vi "Unreserve.vi"(0 "SLSC Remote in":refnum<class "SLSC Remote.lvclass">, 5 "devices":refnum<k21>="$DefaultDevices", 11 "error in (no error)":errorcluster) -> (4 "SLSC Remote out":refnum<class "SLSC Remote.lvclass">, 15 "error out":errorcluster)   [LabVIEW 2016, in "SLSC Interfaces.lvlib" / "SLSC Remote.lvclass"]
uses:
  SLSC Remote.lvclass
  C:/Users/tblair/Documents/Git Projects/SLSC-Interface/Source/SLSC Interface Class/SLSC Interface.lvclass
  <vilib>/NI/JSON Support for LabVIEW/JSON Data Classes/JSON Object/JSON Object.lvclass
  C:/Program Files (x86)/National Instruments/LabVIEW 2016/vi.lib/NI/JSON Support for LabVIEW/JSON Data Classes/JSON Datatype/JSON Null.lvclass
  <vilib>/NI/JSON Support for LabVIEW/JSON Data Classes/JSON Object/New JSON Object (Empty).vi
  <vilib>/NI/JSON Support for LabVIEW/JSON Data Classes/JSON Object/Insert Key Value Pair (Single String).vi
  <vilib>/NI/NI JSONRPC Server Framework/Classes/Server/Format Client Request (Auto-Increment).vi
  <vilib>/httpClient/POSTBuffer.vi
  <vilib>/NI/NI JSONRPC Server Framework/Classes/Server/Parse Response (Object).vi
  <vilib>/NI/NI JSONRPC Server Framework/Classes/Server/JSONRPC Server.lvclass
  <vilib>/httpClient/LabVIEWHTTPClient.lvlib
  <vilib>/NI/JSON Support for LabVIEW/JSON Data Classes/JSON Helper/JSON Helper.lvclass
  C:/Program Files (x86)/National Instruments/LabVIEW 2016/vi.lib/NI/JSON Support for LabVIEW/JSON Data Classes/JSON Structured Type/JSON Structure.lvclass
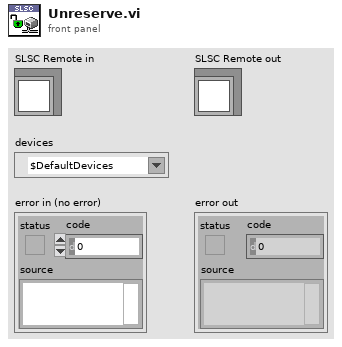
[diagram p1: front panel]
types:
  T1 = typedef "LabVIEWHTTPClient.lvlib/ClientHandle.ctl" = refnum<k1>
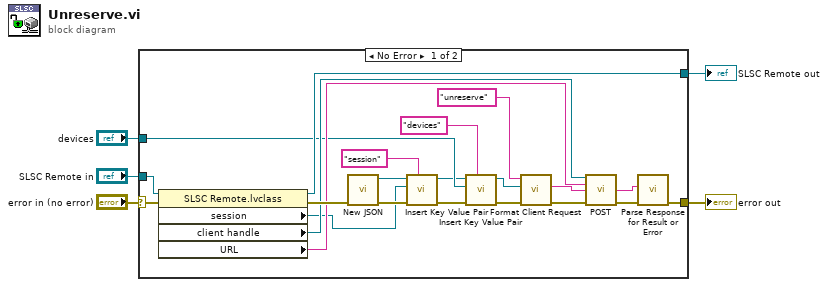
[diagram p0: block diagram]
diagram:
  n1 = case shown="No Error" "error in (no error)" {
    selector: "error in (no error)" -> [w25 w28]
    tunnel: "SLSC Remote in" -> [w27 w29]
    tunnel: [w26 w29] -> w4
    tunnel: [w15 w28] -> w2
    tunnel: "devices" -> [w11 _]
    frame No Error {
      n2 = property class="SLSC Remote.lvclass"(reference=w27, error in=w25) -> (reference out=w26:refnum<class "SLSC Remote.lvclass">, error out=w24:errorcluster, "session"=w10:refnum<k21>, "client handle"=w20:T1, "URL"=w19:string)
      n3 = call-poly <vilib>:"New JSON.vi"("error in (no error)"=w24) -> ("error out"=w23:errorcluster, "JSON Object out"=w6:refnum<class "JSON Object.lvclass">)  [unwired: 9 in]
      n4 = call-poly <vilib>:"Insert Key Value Pair.vi"("key"="session" ("Name"), "error in (no error)"=w23, "value"=w10, "JSON Object in"=w6) -> ("error out"=w14:errorcluster, "JSON Object out"=w7:refnum<class "JSON Object.lvclass">)  [unwired: 5 in, 1 out]
      n5 = call-poly <vilib>:"Insert Key Value Pair.vi"("key"="devices" ("Name"), "error in (no error)"=w14, "value"=w11, "JSON Object in"=w7) -> ("error out"=w12:errorcluster, "JSON Object out"=w13:refnum<class "JSON Object.lvclass">)  [unwired: 5 in, 1 out]
      n6 = call-poly <vilib>:"Format Client Request.vi"("error in (no error)"=w12, "JSON in"=w13, "method"="unreserve") -> ("error out"=w18:errorcluster, "Request String"=w21:string)  [unwired: 7 in]
      n7 = call-poly <vilib>:"POST.vi"("client handle"=w20, "url"=w19, "buffer"=w21, "error in (no error)"=w18) -> ("body"=w17:string, "error out"=w16:errorcluster)  [unwired: 8 in, 2 out]
      n8 = call-poly <vilib>:"Parse Response for Result or Error.vi"("error in"=w16, "Response String In"=w17) -> ("error out"=w15:errorcluster)  [unwired: 7 in, 2 out]
    }
    frame Error {
    }
  }
  "error out" <- w2
  "SLSC Remote out" <- w4
